vi "cost_function_template.vi"(8 "Error In":errorcluster, 10 "Data":variant, 11 "Parameters":dbl[](array[numeric])) -> (0 "Error Out":errorcluster, 3 "Cost":dbl)   [LabVIEW 2016]
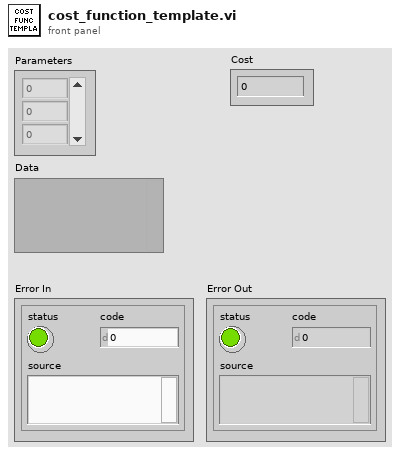
[diagram p1: front panel]
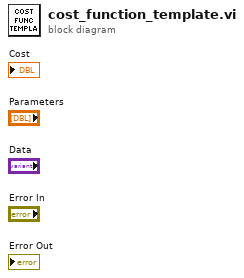
[diagram p0: block diagram]
diagram:
